vi "Register for Recipe Events.vi"(8 "error in (no error)":errorcluster, 11 "Recipe Controller in":refnum<class "Recipe Controller.lvclass">) -> (0 "error out":errorcluster, 1 "Recipe State":refnum<event-registration>, 2 "Recipe Process":refnum<event-registration>, 3 "Recipe Controller out":refnum<class "Recipe Controller.lvclass">)   [LabVIEW 2022 SP3, in "Recipe Controller.lvclass"]
uses:
  Recipe Controller.lvclass
  Recipe Controller.lvclass/Recipe Controller.ctl
  XY Stage/Process Actor/Process Framework/Process State Data/Process State Data.lvclass
  Recipe State Data/Recipe State Data.lvclass
  Recipe State Data/Events.ctl
  XY Stage/Process Actor/Process Framework/Process State Data/Events.ctl
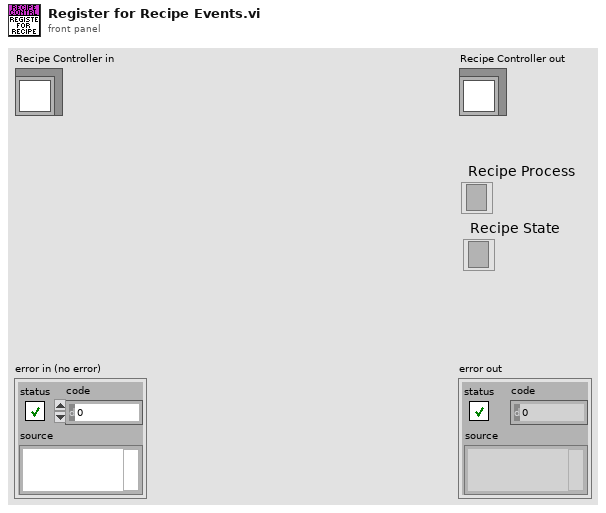
[diagram p1: front panel]
types:
  T1 = typedef "Recipe State Data.lvclass/Events.ctl" = cluster{"Current Recipe Iterations":refnum<user-event>, "Desired Recipe Iterations":refnum<user-event>}
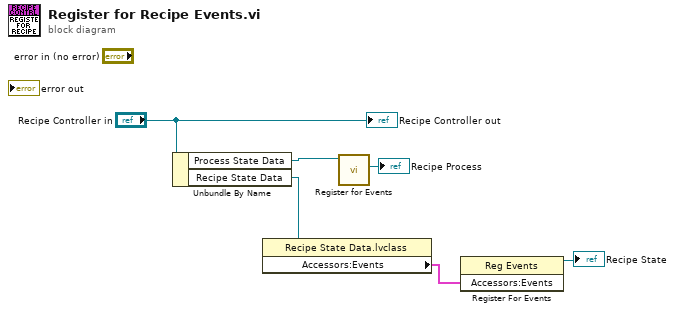
[diagram p0: block diagram]
diagram:
  n1 = Unbundle By Name("Recipe Controller in") -> ("Process State Data"=w5:refnum<data-value>, "Recipe State Data"=w4:refnum<data-value>)
  n2 = property class="Recipe State Data.lvclass"(reference=w4) -> ("Accessors:Events"=w3:T1)  [unwired: 1 in, 2 out]
  n3 = call "Register for Events.vi"("Process State"=w5) -> ("Event Registration Refnum"=→"Recipe Process":refnum<event-registration>)  [unwired: 8 in, 2 out]
  n4 = register-events(w3) -> (reference out=→"Recipe State":refnum<event-registration>)  [unwired: 2 in, 1 out]
  "Recipe Controller out" <- "Recipe Controller in"
